vi "Scripting-Scratchpad.vi"   [LabVIEW 2020]
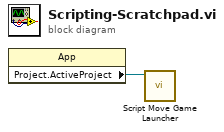
[diagram p0: block diagram]
diagram:
  n1 = property class="App"() -> ("Project.ActiveProject"=w1:refnum<vi>)  [unwired: 2 in, 2 out]
  n2 = call "Script Move Game Launcher.vi"("Project"=w1) -> ()  [unwired: 10 in, 1 out]
